vi "Read one frame from all binary files.vi"(8 "error in (no error)":errorcluster, 9 "Master video's frame number (unity-based)":i32, 10 "Cam Binary Videos (ref)":refnum<file>[](array[refnum]), 11 "Frame numbers & locations in each video file":T3[](array[typedef])) -> (0 "Error out":errorcluster, 2 "Cam Binary Videos (ref)":refnum<file>[](array[refnum]), 3 "Cam videos cluster":T1 {"Vid4 Rel time (ms)" format="%.0f ms"; "Vid3 Rel time (ms)" format="%.0f ms"; "Vid2 Rel time (ms)" format="%.0f ms"; "Vid1 Rel time (ms)" format="%.0f ms"})   [LabVIEW 2013]
uses:
  Typedefs/Number of frames and locations cluster.ctl
  Typedefs/Cam videos cluster.ctl
  <vilib>/vision/Image Controls.llb/IMAQ Image.ctl
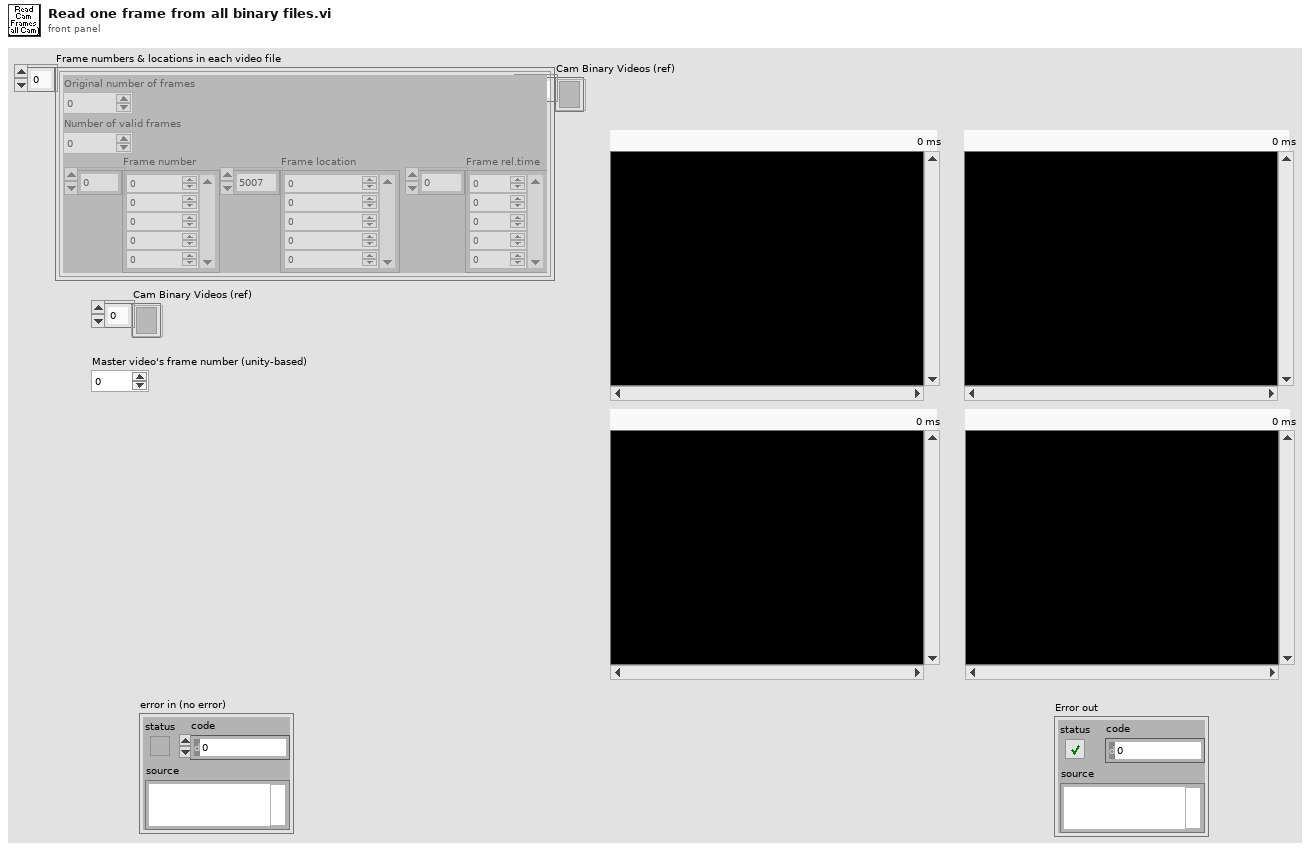
[diagram p1: front panel]
types:
  T1 = typedef "Cam videos cluster.ctl" = cluster{"Vid 1":T2, "Vid 2":T2, "Vid 3":T2, "Vid 4":T2, "Vid1 Rel time (ms)":u32, "Vid2 Rel time (ms)":u32, "Vid3 Rel time (ms)":u32, "Vid4 Rel time (ms)":u32}
  T2 = typedef "IMAQ Image.ctl" = refnum<image>
  T3 = typedef "Number of frames and locations cluster.ctl" = cluster{"Original number of frames":i32, "Number of valid frames":i32, "Frame number":i64[], "Frame location":i64[], "Frame rel.time":i64[]}
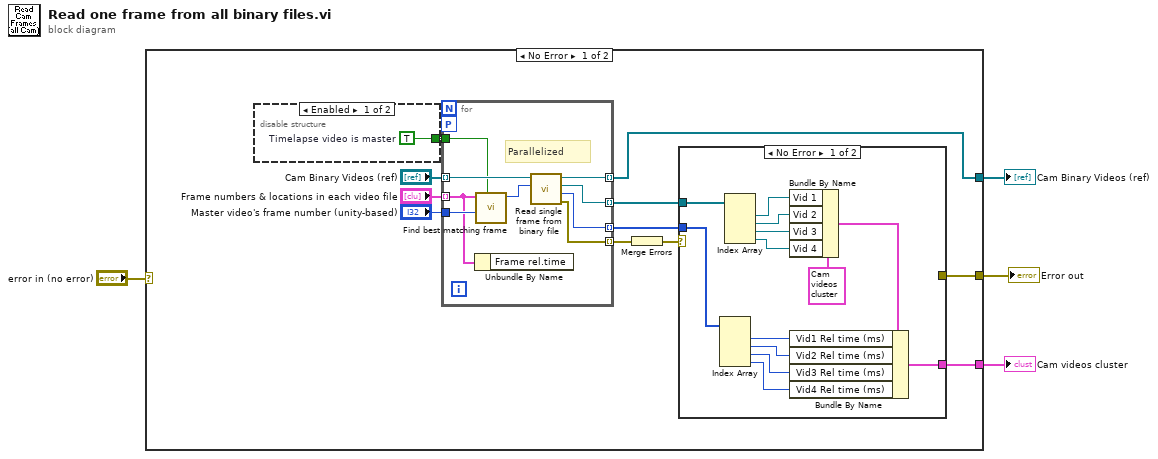
[diagram p0: block diagram]
diagram:
  n1 = case shown="No Error" "error in (no error)" {
    selector: "error in (no error)" -> [_ w40]
    tunnel: [w7 _] -> w4
    tunnel: [w11 _] -> w3
    tunnel: [w8 w40] -> w1
    frame No Error {
      n2 = disable-structure "Diagram Disable Structure" shown="Enabled" {
        disable-tunnel: [w30 _] -> w12
        frame Enabled {
          w30 = TRUE  # Timelapse video is master
        }
        frame Disabled {
        }
      }
      n3 = for {
        tunnel: "Cam Binary Videos (ref)" -> [w37] mode=indexing
        tunnel: "Frame numbers & locations in each video file" -> [w31] mode=indexing
        tunnel: "Master video's frame number (unity-based)" -> [w38]
        tunnel: [w36] -> w7 mode=indexing
        tunnel: w12 -> [w35]
        tunnel: [w34] -> w10 mode=indexing
        tunnel: [w33] -> w9 mode=indexing
        tunnel: [w32] -> w5 mode=indexing
        workers-P: _ -> [_]
        # "Parallelized"
        n4 = Unbundle By Name(w31) -> ()  [unwired: 1 out]
        n5 = call "Find best matching frame.vi"("Timelapse video is master"=w35, "Frame number in master video"=w38, "Cam video frame numbers & locations"=w31) -> ("Nearest frame position in Cam binary file"=w39:i64)  [unwired: 7 in, 1 out]
        n6 = call "Read single frame from binary file.vi"("Frame position in Cam binary file"=w39, "Binary video ref"=w37) -> ("error out"=w32:errorcluster, "Rel time (ms)"=w34:u32, "Image"=w33:T2, "Binary video ref"=w36:refnum<file>)  [unwired: 6 in]
      }
      n7 = Merge Errors(w5) -> (w6:errorcluster)
      n8 = case shown="No Error" w6 {
        selector: w6 -> [_ w29]
        tunnel: [w22 _] -> w11
        tunnel: w10 -> [w21 _]
        tunnel: w9 -> [w16 _]
        tunnel: [_ w29] -> w8
        frame No Error {
          n9 = Index Array(array=w21) -> (element #1=w20:u32, element #2=w19:u32, element #3=w18:u32, element #4=w17:u32)  [unwired: 4 in]
          n10 = Index Array(array=w16) -> (element #1=w27:T2, element #2=w26:T2, element #3=w25:T2, element #4=w24:T2)  [unwired: 4 in]
          n11 = Bundle By Name(cluster=T1 {"Vid 1"=refnum, "Vid 2"=refnum, "Vid 3"=refnum, "Vid 4"=refnum, "Vid1 Rel time (ms)"=0, "Vid2 Rel time (ms)"=0, "Vid3 Rel time (ms)"=0, "Vid4 Rel time (ms)"=0} ("Cam videos cluster"), "Vid 1"=w27, "Vid 2"=w26, "Vid 3"=w25, "Vid 4"=w24) -> (w23:T1)
          n12 = Bundle By Name(cluster=w23, "Vid1 Rel time (ms)"=w20, "Vid2 Rel time (ms)"=w19, "Vid3 Rel time (ms)"=w18, "Vid4 Rel time (ms)"=w17) -> (w22:T1)
        }
        frame Error {
        }
      }
    }
    frame Error {
    }
  }
  "Cam Binary Videos (ref)" <- w4
  "Cam videos cluster" <- w3
  "Error out" <- w1
